vi "Create Map of Parameter Names.vi"(8 "error in (no error)":errorcluster, 11 "FPGA Interface in":refnum<class "FPGA Interface.lvclass">) -> (0 "error out":errorcluster, 2 "Parameters":map{string, string[]}(c390), 3 "FPGA Interface out":refnum<class "FPGA Interface.lvclass">)   [LabVIEW 2026, in "TALOS.lvlib" / "Interfaces.lvlib" / "FPGA Interface.lvclass"]
uses:
  FPGA Interface.lvclass
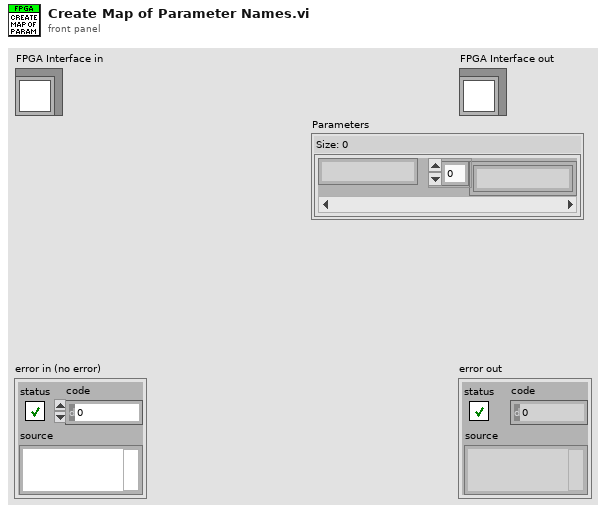
[diagram p1: front panel]
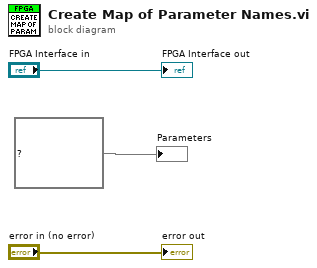
[diagram p0: block diagram]
diagram:
  "error out" <- "error in (no error)"
  "FPGA Interface out" <- "FPGA Interface in"
  "Parameters" <- map{string, string[]} {} ("Parameters")
